vi "ConfigureRobotProfile.vi"(0 "Selected Robot":i32) -> ()   [LabVIEW 2020]
doc: "Uses robot profile information to determine which sensors should be bypassed"
uses:
  robotprofiles.vi
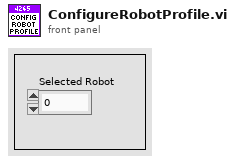
[diagram p1: front panel]
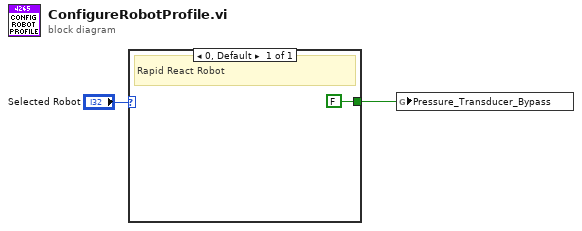
[diagram p0: block diagram]
diagram:
  n1 = case shown="0, Default" "Selected Robot" {
    tunnel: [FALSE ("Pressure_Transducer_Bypass")] -> w1
    frame 0, Default {
      # "Rapid React Robot"
    }
  }
  n2 = global write "robotprofiles.vi" "Pressure_Transducer_Bypass"(w1) -> ()
